vi "Auto Rotate By Gyro.vi"(0 "Gyro Name":string, 1 "Wanted Angle":dbl) -> (2 "Left Stick Value":dbl, 3 "Right Stick Value":dbl, 4 "Completed?":bool)   [LabVIEW 2012]
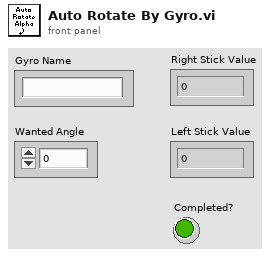
[diagram p1: front panel]
types:
  T1 = typedef "WPI_GyroDevRef.ctl" = cluster{"DevStatus":errorcluster, "Analog Module":T2, "Analog Channel":T3, "Offset":dbl, "Gain (VoltsPerDegree/Second)":dbl}
  T2 = typedef "FPGA_TypedefAnalogModule.ctl" = enum16{"Analog Module 1", "Analog Module 2"}
  T3 = typedef "FPGA_AIChannel.ctl" = enum8{"AI 1", "AI 2", "AI 3", "AI 4", "AI 5", "AI 6", "AI 7", "AI 8", "Invalid"}
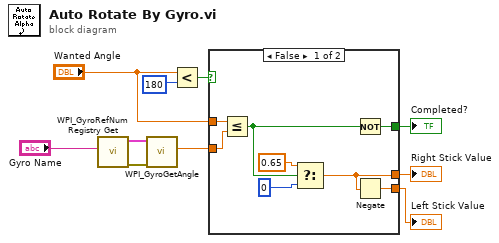
[diagram p0: block diagram]
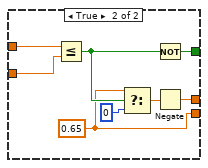
[diagram p2: hidden frame]
diagram:
  n1 = call <vilib>:"WPI_GyroRefNum Registry Get.vi"("refnum name"="Gyro Name") -> ("error out"=w8:errorcluster, "GyroDevRef"=w9:T1)  [unwired: 9 in]
  n2 = call <vilib>:"WPI_GyroGetAngle.vi"("error in (no error)"=w8, "GyroDevRef"=w9) -> ("Angle"=w5:dbl)  [unwired: 6 in, 3 out]
  n3 = Less?(x="Wanted Angle", y=180) -> (x < y?=w6:bool)
  n4 = case shown="False" w6 {
    tunnel: w5 -> [w17 w20]
    tunnel: [w18 w22] -> w4
    tunnel: [w14 w23] -> w3
    tunnel: "Wanted Angle" -> [w16 w21]
    tunnel: [w12 w19] -> w1
    frame False {
      n5 = Less Or Equal?(x=w16, y=w17) -> (x <= y?=w11:bool)
      n6 = Select(t=0.65, s=w11, f=0) -> (s? t:f=w14:dbl)
      n7 = Not(x=w11) -> (.not. x?=w12:bool)
      n8 = Negate(x=w14) -> (-x=w18:dbl)
    }
    frame True {
      w22 = 0.65
      n9 = Less Or Equal?(x=w21, y=w20) -> (x <= y?=w24:bool)
      n10 = Select(t=w22, s=w24, f=0) -> (s? t:f=w26:dbl)
      n11 = Not(x=w24) -> (.not. x?=w19:bool)
      n12 = Negate(x=w26) -> (-x=w23:dbl)
    }
  }
  "Right Stick Value" <- w3
  "Left Stick Value" <- w4
  "Completed?" <- w1
